vi "fgv_scout_serial.vi"(7 "cmd":enum16{"ini", "write", "read", "close"}(ring), 8 "error in":errorcluster, 9 "Frame ID":u8, 10 "control-val":T1) -> (0 "error out":errorcluster, 2 "read buffer n":u32, 3 "read data":string)   [LabVIEW 2019]
uses:
  <vilib>/Instr/_visa.llb/VISA Configure Serial Port (Instr).vi
  Subvi/global_setting.vi
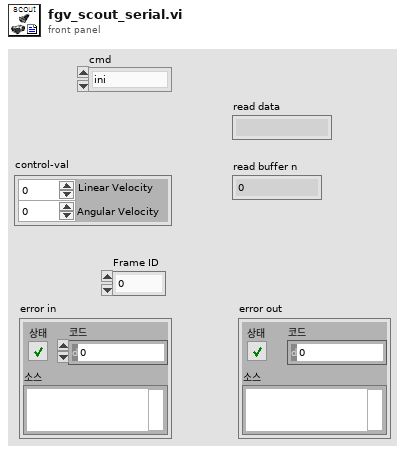
[diagram p1: front panel]
types:
  T1 = cluster{"Linear Velocity":dbl, "Angular Velocity":dbl}
  T2 = typedef "IMAQdx.ctl" = refnum<k21>
  T3 = typedef "system_hw.ctl" = cluster{"AGV":enum16{"none", "ERP42", "ERP42mini", "Scout", "Ycar"}, "Lidar 1":enum16{"none", "VLP16", "TIM571", "RPLidar A2", "RPLidar A3"}, "Lidar 2":enum16{"none", "VLP16", "TIM571", "RPLidar A2", "RPLidar A3"}, "GPS":enum16{"none", "F9P", "M8P", "PwrPak7", "19X HVS"}, "Camera":enum16{"none", "C920", "C922", "GT1290C", "MS LifeCam"}, "Joystick":enum16{"none", "joystick"}}
  T4 = typedef "joystick cfg.ctl" = cluster{"Type":enum16{"Logitech F710", "Xbox"}, "steer limit":cluster{"min":dbl, "max":dbl, "scale":dbl, "offset":dbl}, "speed limit":cluster{"min":dbl, "max":dbl, "pwm max":dbl}, "ID":i32, "joystick max":dbl}
  T5 = cluster{"VLP16 cfg":cluster{"h range":cluster{i16, i16}, "v range":cluster{i8, i8}}, "TIM571 cfg":cluster{"IP":string, "h range":cluster{i16, i16}}, "AGV cfg":cluster{"Port":refnum<visa-resource-name>, "speed limits":cluster{"limit_linear-v":dbl, "limit_angular-v":dbl}, "limits":cluster{"speed limits":cluster{"max":dbl, "min":dbl}, "steer limits":cluster{"max":dbl, "min":dbl}}}, "GPS cfg":cluster{"PwrPak7 Port":refnum<visa-resource-name>, "heading select":string, "mode select":string[]}, "PID cfg":cluster{"PID gains":cluster{"proportional gain (Kc)":dbl, "integral time (Ti, min)":dbl, "derivative time (Td, min)":dbl}, "PID limits":cluster{"output high":dbl, "output low":dbl}, "dt pid":u32}, "Lookahead cfg":cluster{"lookahead pts n":dbl, "lookahead distance":dbl}, "Obstacle limit range":cluster{"RL range":dbl, "Point limit":u16}, "State machine parameter":cluster{"angle adjust limit":dbl}, "waypoint group":cluster{"Waypoint array":cluster{"sel":bool, "inv":bool, "path":path}[]}, "State machine cfg":cluster{" turn angular speed":dbl, "move linear speed":dbl, "decrease factor linear speed":dbl, "adjust angle margin":dbl}, "camera cfg":cluster{"Port":T2, "Camera file":path}, "ROI-clamp":cluster{"Global Rectangle":i32[], "Contours":cluster{"Contour Type":u32, "ROI Type":u32, "Points":i32[]}[]}, "x-center":dbl, "Image Size":cluster{"x":i32, "y":i32}, "Angle deg":sgl, "Vison cfg":cluster{"Clamp Settings":cluster{"Contrast":i32, "Filter width":i32, "Steepness":i32, "Subsampling Ratio":u32, "Show Search Area":bool, "Show Search Lines":bool, "Show Edges Found":bool, "Show Result":bool}, "Range":cluster{"Lower value":sgl, "Upper value":sgl}, "N of Erosion 1":i32, "N of Erosion 2":i32}, "RPLidar cfg":cluster{"port":refnum<visa-resource-name>, "dt":u32, "update":u8, "speed":u16, "rate ":u32}, "HW info":T3, "Joystick cfg":T4}
  T6 = cluster{"Port":refnum<visa-resource-name>, "speed limits":cluster{"speed-limit":dbl, "steer-limit":dbl}, "limits":cluster{"speed limits":cluster{"max":dbl, "min":dbl}, "steer limits":cluster{"max":dbl, "min":dbl}}}
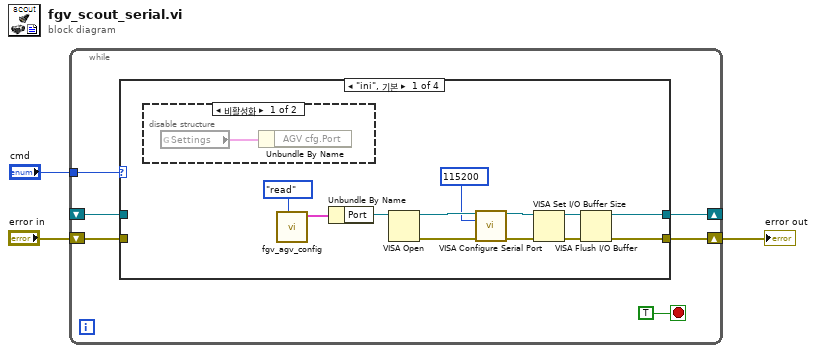
[diagram p0: block diagram]
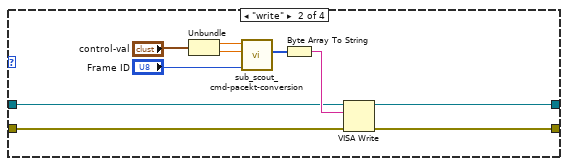
[diagram p3: hidden frame]
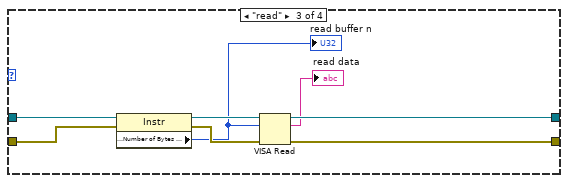
[diagram p4: hidden frame]
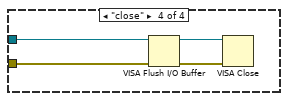
[diagram p5: hidden frame]
diagram:
  n1 = while {
    tunnel: "cmd" -> [w8]
    shift-right: [w7] -> w2
    shift-left: "error in" -> [w5]
    shift-right: [w6] -> _
    shift-left: _ -> [w4]
    stop <- TRUE stop-if-true
    n2 = case shown="\"ini\", 기본" w8 {
      tunnel: [w13 w29 w36 _] -> w7
      tunnel: [w14 w30 w35 _] -> w6
      tunnel: w5 -> [_ w28 w38 w42]
      tunnel: w4 -> [_ w27 w37 w41]
      frame "ini", Default {
        n3 = disable-structure shown="비활성화" {
          frame Disabled {
            n4 = global read "global_setting.vi" "Settings"() -> (w22:T5)
            n5 = Unbundle By Name(w22) -> ()  [unwired: 1 out]
          }
          frame Enabled {
          }
        }
        n6 = call "fgv_agv_config.vi"("cmd"=enum16{"read", "write"}."read") -> ("AGV cfg out"=w11:T6)  [unwired: 9 in, 1 out]
        n7 = Unbundle By Name(w11) -> ("Port"=w10:refnum<visa-resource-name>)
        n8 = VISA Open(VISA resource name=w10) -> (VISA resource name=w17:refnum<visa-resource-name>, error out=w16:errorcluster)  [unwired: 4 in]
        n9 = call-poly "VISA Configure Serial Port"("VISA resource name"=w17, "baud rate (9600)"=u32 115200, "error in (no error)"=w16) -> ("VISA resource name out"=w20:refnum<visa-resource-name>, "error out"=w19:errorcluster)  [unwired: 11 in]
        n10 = VISA Set I/O Buffer Size(VISA resource name=w20, error in (no error)=w19) -> (VISA resource name out=w18:refnum<visa-resource-name>, error out=w21:errorcluster)  [unwired: 2 in]
        n11 = VISA Flush I/O Buffer(VISA resource name=w18, error in (no error)=w21) -> (VISA resource name out=w14:refnum<visa-resource-name>, error out=w13:errorcluster)  [unwired: 1 in]
      }
      frame "write" {
        n12 = Unbundle("control-val") -> ("Linear Velocity"=w24:dbl, "Angular Velocity"=w25:dbl)
        n13 = call "sub_scout_cmd-pacekt-conversion.vi"("Frame ID"="Frame ID", "Angular Velocity"=w25, "Linear Velocity"=w24) -> ("CMD"=w31:u8[])  [unwired: 8 in]
        n14 = Byte Array To String(unsigned byte array=w31) -> (string=w32:string)
        n15 = VISA Write(VISA resource name=w27, write buffer=w32, error in (no error)=w28) -> (VISA resource name out=w30:refnum<visa-resource-name>, error out=w29:errorcluster)  [unwired: 1 out]
      }
      frame "read" {
        n16 = property class="Instr"(reference=w37, error in=w38) -> (reference out=w39:refnum<visa-resource-name>, error out=w40:errorcluster, "Serial Settings:Number of Bytes at Serial Port"=w34:u32)
        "read buffer n" <- w34
        n17 = VISA Read(VISA resource name=w39, byte count=w34, error in (no error)=w40) -> (VISA resource name out=w35:refnum<visa-resource-name>, read buffer=→"read data":string, error out=w36:errorcluster)  [unwired: 1 out]
      }
      frame "close" {
        n18 = VISA Flush I/O Buffer(VISA resource name=w41, error in (no error)=w42) -> (VISA resource name out=w43:refnum<visa-resource-name>, error out=w44:errorcluster)  [unwired: 1 in]
        n19 = VISA Close(VISA resource name=w43, error in (no error)=w44) -> ()  [unwired: 1 out]
      }
    }
  }
  "error out" <- w2
